vi "Build old.vi"(7 "channel blocks":T1[](array[typedef]) {"dst buffer offset" format="%d bytes"; "src buffer offset" format="%d bytes"}, 8 "error in (no error)":errorcluster, 9 "dst Buffer":refnum<class "Buffer.lvclass">, 10 "src Buffer":refnum<class "DBL Pointer.lvclass">, 11 "Buffer Converter in":refnum<class "Buffer Converter.lvclass">) -> (0 "error out":errorcluster, 3 "Buffer Converter out":refnum<class "Buffer Converter.lvclass">)   [LabVIEW 2017, in "DSF Core.lvlib" / "Buffer Converter.lvclass"]
uses:
  Buffer Converter.lvclass
  Buffer/Buffer.lvclass
  Pointer/DBL Pointer.lvclass
  DSF Configuration API/Public/Controls/DSF Data Type.ctl
  DSF Core.lvlib
  DSF Configuration API/Public/Controls/DSF Engine Channel Configuration.ctl
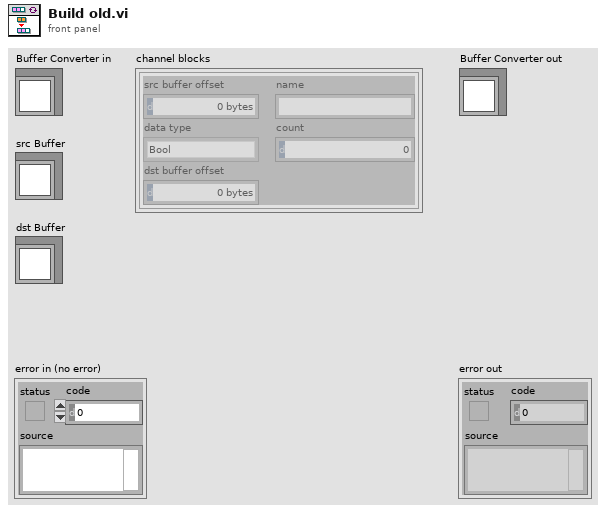
[diagram p1: front panel]
types:
  T1 = typedef "DSF Core.lvlib/DSF Engine Channel Configuration.ctl" = cluster{"src buffer offset":u64, "name":string, "data type":T2, "count":u64, "dst buffer offset":u64}
  T2 = typedef "DSF Core.lvlib/DSF Data Type.ctl" = enum8{"Bool", "SGL", "DBL", "I8", "I16", "I32", "I64", "U8", "U16", "U32", "U64"}
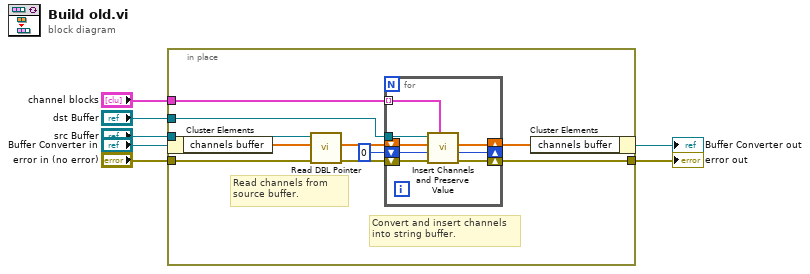
[diagram p0: block diagram]
diagram:
  n1 = in-place {
    in-place-border: [w17] -> w7
    in-place-border: "channel blocks" -> [w16]
    in-place-border: "src Buffer" -> [w15]
    in-place-border: "error in (no error)" -> [w14]
    in-place-border: "dst Buffer" -> [w10]
    # "Read channels from source buffer."
    # "Convert and insert channels into string buffer."
    n2 = in-place-cluster #1("Buffer Converter in") -> ("channels buffer"=w9:dbl[])
    n3 = call "Read DBL Pointer.vi"("error in (no error)"=w14, "buffer in"=w9, "DBL Pointer in"=w15) -> ("error out"=w13:errorcluster, "buffer out"=w12:dbl[])  [unwired: 6 in, 1 out]
    n4 = for {
      shift-right: [w23] -> w8
      shift-left: w12 -> [w24]
      shift-right: [w22] -> w17
      shift-left: w13 -> [w25]
      tunnel: w10 -> [w21]
      tunnel: w16 -> [w20] mode=indexing
      shift-right: [w19] -> _
      shift-left: u64 0 ("channels buffer index in") -> [w18]
      n5 = call "Insert Channels and Preserve Value.vi"("channel block"=w20, "error in (no error)"=w25, "channels buffer index in"=w18, "channels buffer in"=w24, "Buffer in"=w21) -> ("error out"=w22:errorcluster, "channels buffer index out"=w19:u64, "channels buffer out"=w23:dbl[])  [unwired: 3 in, 1 out]
    }
    n6 = in-place-cluster #1("channels buffer"=w8) -> (→"Buffer Converter out":refnum<class "Buffer Converter.lvclass">)
  }
  "error out" <- w7
